vi "Request Chamber State.vi"(6 "wait for reply (T)":bool=TRUE, 8 "error in (no error)":errorcluster, 11 "Thermal Chamber Controller In":refnum<class "Thermal Chamber Controller.lvclass">) -> (0 "error out":errorcluster, 1 "timed out?":bool, 2 "Chamber Status Reply Payload":T1={"Actual Temperature"=0.0, "Temperature Set Point"=0.0, "Temperature Ramp Rate"=0.0, "Heater State"=enum."Heater Enabled"}, 3 "Thermal Chamber Controller Out":refnum<class "Thermal Chamber Controller.lvclass">)   [LabVIEW 2020, in "Thermal Chamber Controller.lvclass"]
uses:
  Thermal Chamber Controller.lvclass
  C:/Program Files (x86)/National Instruments/LabVIEW 2020/vi.lib/Astemes/Triarc Framework/Process/Process.lvclass
  Chamber State.ctl
  Private/Heater State.ctl
  <vilib>/Astemes/Triarc Framework/Process/Process.lvclass/Process.ctl
  <vilib>/Astemes/Triarc Framework/Process/Private/SubVIs/Handle Debug Data.vi
  <vilib>/Astemes/Triarc Framework/Process/Protected/Messaging/Async Request Message.vi
  <vilib>/Astemes/Triarc Framework/Synchronous Request Callback/Synchronous Request Callback.lvclass
  C:/Program Files (x86)/National Instruments/LabVIEW 2020/vi.lib/Astemes/Triarc Framework/Callback/Callback.lvclass
  <vilib>/Utility/error.llb/Error Cluster From Error Code.vi
  <vilib>/Astemes/Triarc Framework/Process/Public/Lifecycle/Get Lifecycle State.vi
  <vilib>/Astemes/Triarc Framework/Synchronous Request Callback/Create.vi
  <vilib>/Astemes/Triarc Framework/Process/Private/SubVIs/Wait for Response Message.vi
  <vilib>/Astemes/Triarc Framework/Callback/Callback.lvclass
  <vilib>/Astemes/Triarc Framework/Process/Process.lvclass
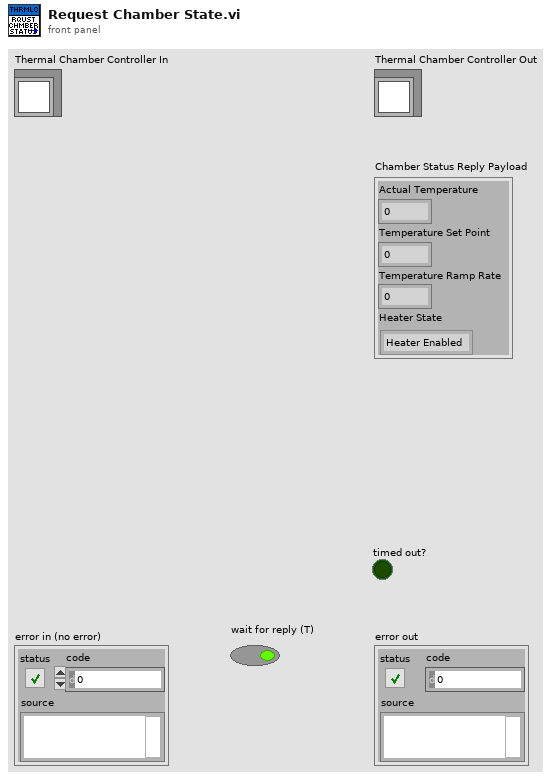
[diagram p1: front panel]
types:
  T1 = typedef "Thermal Chamber Controller.lvclass/Chamber State.ctl" = cluster{"Actual Temperature":dbl, "Temperature Set Point":dbl, "Temperature Ramp Rate":dbl, "Heater State":T2}
  T2 = typedef "Thermal Chamber Controller.lvclass/Heater State.ctl" = enum16{"Heater Disabled", "Heater Enabled"}
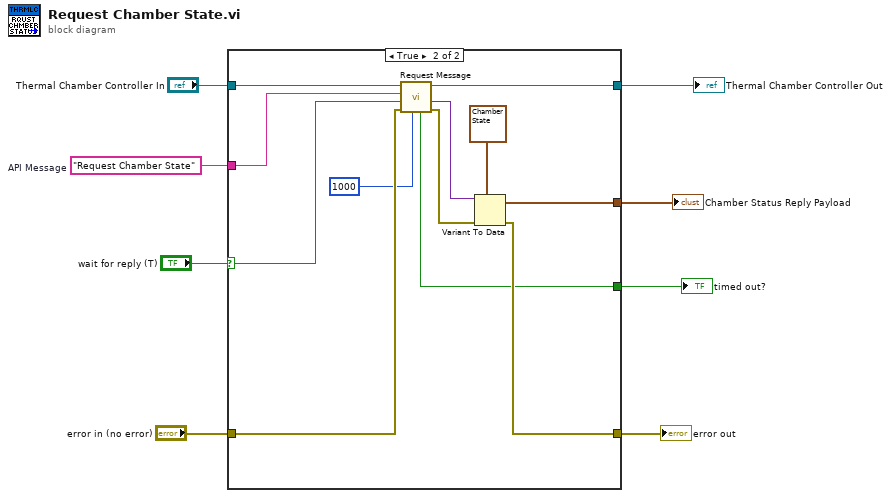
[diagram p0: block diagram]
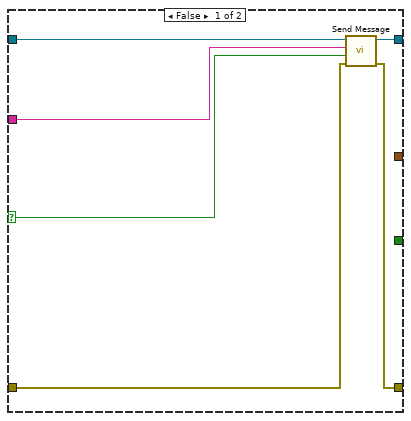
[diagram p2: hidden frame]
diagram:
  w3 = "Request Chamber State"  # API Message
  n1 = case shown="True" "wait for reply (T)" {
    selector: "wait for reply (T)" -> [w9 w15]
    tunnel: [w14 w23] -> w8
    tunnel: [w13 w18] -> w7
    tunnel: "error in (no error)" -> [w12 w24]
    tunnel: "Thermal Chamber Controller In" -> [w11 w26]
    tunnel: w3 -> [w10 w25]
    tunnel: [_ w21] -> w2
    tunnel: [_ w17] -> w1
    frame False {
      n2 = call <vilib>:"Send Message.vi"("error in (no error)"=w12, "Message Data"=w9, "Message"=w10, "Process In"=w11) -> ("error out"=w13:errorcluster, "Process Out"=w14:refnum<class "Thermal Chamber Controller.lvclass">)  [unwired: 6 in]
    }
    frame True {
      n3 = call <vilib>:"Request Message.vi"("timeout in ms (-1)"=1000, "error in (no error)"=w24, "Request Message Data"=w15, "Request Message"=w25, "Process In"=w26) -> ("error out"=w19:errorcluster, "Response Message Data"=w20:variant, "Process Out"=w23:refnum<class "Thermal Chamber Controller.lvclass">, "Timed out?"=w17:bool)  [unwired: 2 in, 1 out]
      n4 = Variant To Data(error in=w19, type=T1 {"Actual Temperature"=0.0, "Temperature Set Point"=0.0, "Temperature Ramp Rate"=0.0, "Heater State"=enum."Heater Enabled"} ("Chamber Status Reply Payload"), Variant=w20) -> (data=w21:T1, error out=w18:errorcluster)
    }
  }
  "error out" <- w7
  "Thermal Chamber Controller Out" <- w8
  "timed out?" <- w1
  "Chamber Status Reply Payload" <- w2
